vi "Move Right Axis.vi"(3 "Make Vertical":bool, 4 "Side":T1=enum."right", 5 "Label":string="Z", 6 "Wait Time":dbl, 8 "error in":errorcluster, 9 "Speed":dbl=25.0, 10 "Value":dbl, 11 "Location":string="Z") -> (0 "error out":errorcluster)   [LabVIEW 2013]
uses:
  ROS/Code/SubVIs/BaxterSide.ctl
  Arm Globals.vi
  Prim/Fwd Kenimatics - array.vi
  <vilib>/Analysis/Matrix/Numeric/Multiply/Multiply - RM,RM.vi
  <vilib>/Analysis/Matrix/NI_Matrix.lvlib
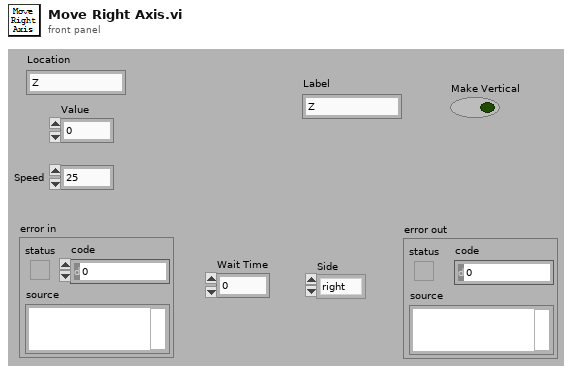
[diagram p1: front panel]
types:
  T1 = typedef "BaxterSide.ctl" = enum16{"left", "right"}
  T2 = typedef "NI_Matrix.lvlib/RealMatrix.ctl" = dbl[][]
  T3 = cluster{"X":dbl, "Y":dbl, "Z":dbl, "Roll":dbl, "Pitch":dbl, "Yaw":dbl}
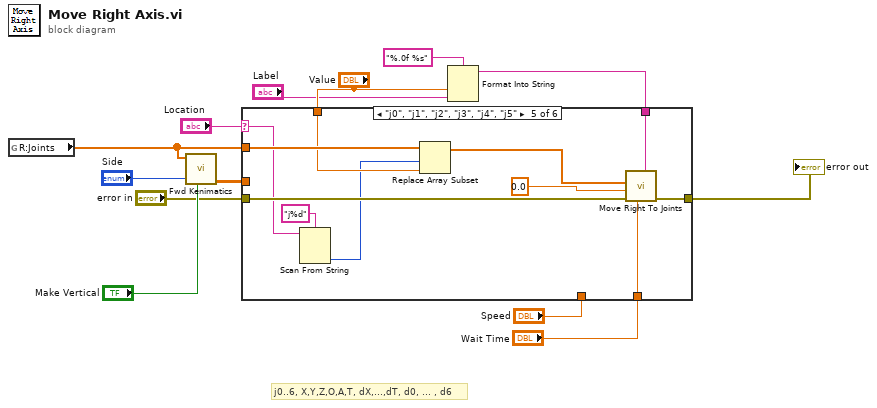
[diagram p0: block diagram]
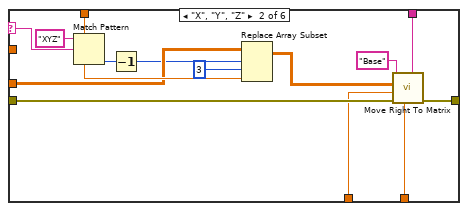
[diagram p3: hidden frame]
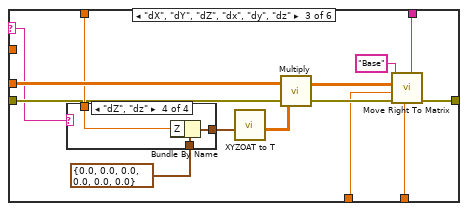
[diagram p4: hidden frame]
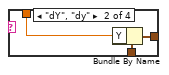
[diagram p6: hidden frame]
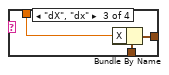
[diagram p7: hidden frame]
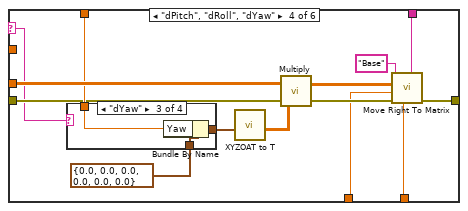
[diagram p8: hidden frame]
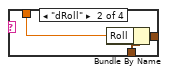
[diagram p10: hidden frame]
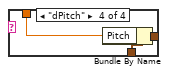
[diagram p11: hidden frame]
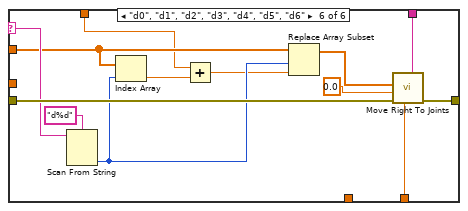
[diagram p12: hidden frame]
diagram:
  # "j0..6, X,Y,Z,O,A,T, dX,...,dT, d0, ... , d6"
  n1 = global read "Arm Globals.vi" "R:Joints"() -> (w1:dbl[])
  n2 = call-poly "Fwd Kenimatics.vi"("Make Vertical"="Make Vertical", "Side"="Side", "Joints"=w1) -> ("Matrix"=w10:T2)  [unwired: 7 in, 1 out]
  n3 = Format Into String(format string="%.0f %s" ("Label"), "Value", "Label") -> (resulting string=w7:string)  [unwired: 2 in, 1 out]
  n4 = case shown="\"j0\", \"j1\", \"j2\", \"j3\", \"j4\", \"j5\"" "Location" {
    selector: "Location" -> [_ w19 w30 w53 w79 w94]
    tunnel: "Value" -> [_ w27 w37 w60 w84 w89]
    tunnel: w10 -> [_ w26 w38 w61 _ _]
    tunnel: w1 -> [_ _ _ _ w85 w92]
    tunnel: w7 -> [_ w23 w32 w55 w76 w87]
    tunnel: "error in" -> [w14 w22 w35 w58 w80 w95]
    tunnel: [w14 w21 w31 w54 w81 w96] -> w6
    tunnel: "Speed" -> [_ w20 w33 w56 _ _]
    tunnel: "Wait Time" -> [_ w15 w29 w52 w75 w86]
    frame Default {
    }
    frame "X", "Y", "Z" {
      n5 = Match Pattern(string="XYZ", regular expression=w19) -> (offset past match=w17:i32)  [unwired: 1 in, 3 out]
      n6 = Decrement(x=w17) -> (x-1=w16:i32)
      n7 = Replace Array Subset(array=w26, new element=w27, index (row)=w16, index (col)=3 ("disabled index (row)")) -> (w25:T2)
      n8 = call "Move Right To Matrix.vi"("Label"=w23, "Wait Time"=w15, "error in"=w22, "Speed (mm/s)"=w20, "Offset"=w25, "Location"="Base") -> ("error out"=w21:errorcluster)  [unwired: 5 in]
    }
    frame "dX", "dY", "dZ", "dx", "dy", "dz" {
      n9 = case shown="\"dZ\", \"dz\"" w30 {
        tunnel: [w42 w45 w48 w51] -> w41
        tunnel: T3 {"X"=0.0, "Y"=0.0, "Z"=0.0, "Roll"=0.0, "Pitch"=0.0, "Yaw"=0.0} ("XYZOAT") -> [w42 w44 w47 w50]
        tunnel: w37 -> [_ w43 w46 w49]
        frame Default {
        }
        frame "dY", "dy" {
          n10 = Bundle By Name(cluster=w44, "Y"=w43) -> (w45:T3)
        }
        frame "dX", "dx" {
          n11 = Bundle By Name(cluster=w47, "X"=w46) -> (w48:T3)
        }
        frame "dZ", "dz" {
          n12 = Bundle By Name(cluster=w50, "Z"=w49) -> (w51:T3)
        }
      }
      n13 = call "XYZOAT to T.vi"("XYZOAT"=w41) -> ("T"=w39:T2)  [unwired: 10 in]
      n14 = call-poly <vilib>:"Multiply.vi"("Real Matrix B"=w39, "Real Matrix A"=w38) -> ("A * B"=w34:T2)
      n15 = call "Move Right To Matrix.vi"("Label"=w32, "Wait Time"=w29, "error in"=w35, "Speed (mm/s)"=w33, "Offset"=w34, "Location"="Base") -> ("error out"=w31:errorcluster)  [unwired: 5 in]
    }
    frame "dPitch", "dRoll", "dYaw" {
      n16 = case shown="\"dYaw\"" w53 {
        tunnel: [w65 w68 w71 w74] -> w64
        tunnel: T3 {"X"=0.0, "Y"=0.0, "Z"=0.0, "Roll"=0.0, "Pitch"=0.0, "Yaw"=0.0} ("XYZOAT") -> [w65 w67 w70 w73]
        tunnel: w60 -> [_ w66 w69 w72]
        frame Default {
        }
        frame "dRoll" {
          n17 = Bundle By Name(cluster=w67, "Roll"=w66) -> (w68:T3)
        }
        frame "dYaw" {
          n18 = Bundle By Name(cluster=w70, "Yaw"=w69) -> (w71:T3)
        }
        frame "dPitch" {
          n19 = Bundle By Name(cluster=w73, "Pitch"=w72) -> (w74:T3)
        }
      }
      n20 = call "XYZOAT to T.vi"("XYZOAT"=w64) -> ("T"=w62:T2)  [unwired: 10 in]
      n21 = call-poly <vilib>:"Multiply.vi"("Real Matrix B"=w62, "Real Matrix A"=w61) -> ("A * B"=w57:T2)
      n22 = call "Move Right To Matrix.vi"("Label"=w55, "Wait Time"=w52, "error in"=w58, "Speed (mm/s)"=w56, "Offset"=w57, "Location"="Base") -> ("error out"=w54:errorcluster)  [unwired: 5 in]
    }
    frame "j0", "j1", "j2", "j3", "j4", "j5" {
      n23 = Scan From String(format string="j%d", input string=w79) -> (output 1=w77:i32)  [unwired: 3 in, 3 out]
      n24 = Replace Array Subset(array=w85, new element=w84, index=w77) -> (w83:dbl[])
      n25 = call "Move Right To Joints.vi"("Label"=w76, "Wait (s)"=w75, "error in"=w80, "time"=0.0, "Goal"=w83) -> ("error out"=w81:errorcluster)  [unwired: 6 in]
    }
    frame "d0", "d1", "d2", "d3", "d4", "d5", "d6" {
      n26 = Scan From String(format string="d%d", input string=w94) -> (output 1=w91:i32)  [unwired: 3 in, 3 out]
      n27 = Index Array(array=w92, index=w91) -> (element=w90:dbl)
      n28 = Add(x=w89, y=w90) -> (x+y=w88:dbl)
      n29 = Replace Array Subset(array=w92, new element=w88, index=w91) -> (w98:dbl[])
      n30 = call "Move Right To Joints.vi"("Label"=w87, "Wait (s)"=w86, "error in"=w95, "time"=0.0, "Goal"=w98) -> ("error out"=w96:errorcluster)  [unwired: 6 in]
    }
  }
  "error out" <- w6
